vi "Read Frame Nr.vi"(8 "error in (no error)":errorcluster, 11 "HIJ Vision Camera App in":refnum<class "HIJ Vision Camera App.lvclass">) -> (0 "error out":errorcluster, 2 "Frame Nr":i32, 3 "HIJ Vision Camera App out":refnum<class "HIJ Vision Camera App.lvclass">)   [LabVIEW 2020, in "HIJ Vision Camera App.lvlib" / "HIJ Vision Camera App.lvclass"]
uses:
  HIJ Vision Camera App.lvclass
  HIJ Vision Camera App.lvclass/HIJ Vision Camera App.ctl
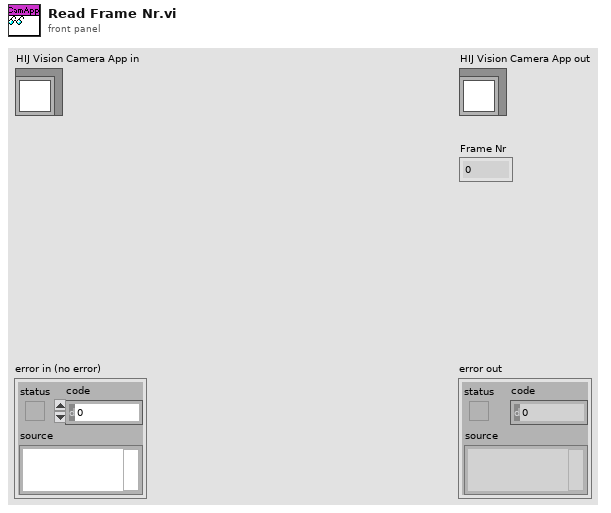
[diagram p1: front panel]
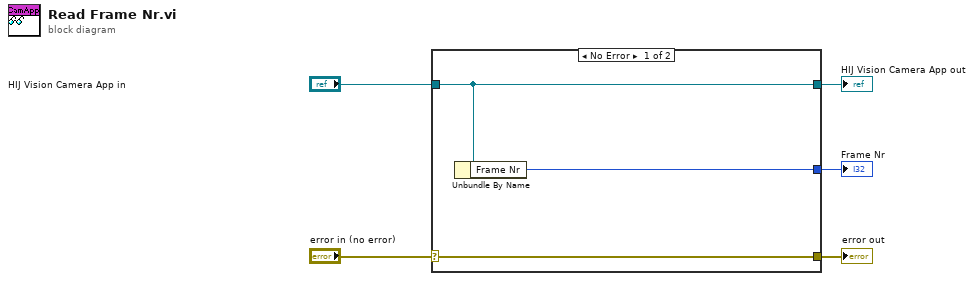
[diagram p0: block diagram]
diagram:
  n1 = case shown="No Error" "error in (no error)" {
    selector: "error in (no error)" -> [w8 w9]
    tunnel: [w8 w9] -> w4
    tunnel: [w7 w10] -> w2
    tunnel: "HIJ Vision Camera App in" -> [w7 w10]
    tunnel: [w6 _] -> w1
    frame No Error {
      n2 = Unbundle By Name(w7) -> ("Frame Nr"=w6:i32)
    }
    frame Error {
    }
  }
  "error out" <- w4
  "HIJ Vision Camera App out" <- w2
  "Frame Nr" <- w1
